vi "Tesina_Frullo_Corrado.vi"() -> ()   [LabVIEW 2021]
uses:
  <vilib>/express/express analysis/Spectral/XNode/ExpressSpectralMeasurementsBlockNode.xnode
  <vilib>/express/express analysis/Spectral/Block/exnSpectralBlock spectral measurements RMS poly.vi
  <vilib>/express/express analysis/Spectral/Block/exnSpectralBlock spectral measurements RMS array WFM.vi
  <vilib>/express/express analysis/Spectral/Block/exnSpectralBlock spectral measurements RMS DDT.vi
panel:
  in  "Lower Cut-Off (Hz)":dbl=100.0 caption="Lower Cut-Off"
  out "Originale":bool
  out "Filtrato":bool
  out "Caricamento...":i32(slide) scale=0.0..4.0
  in  "Vuoi ascoltare il campione filtrato?":bool
  out "FFT - (RMS) [filtrato]":dynamicdata(graph)
  out "Time-domain [filtrato]":dynamicdata(graph)
  in  "Vuoi filtrare il campione?":bool
  out "Quando il led si accende, preparati a registrare!":bool
  out "FFT - (RMS)":cluster{"f0":dbl, "df":dbl, "magnitude":dbl[]}[](graph)
  out "Time-domain":waveform(dbl)[](graph)
  in  "Vuoi riascoltare il campione caricato?":bool
  in  "Carica file da analizzare [.wav]":path
  in  "1) Vuoi registrare un campione o analizzarne uno già salvato?":bool
  in  "Salva file [.wav]":path
  in  "Vuoi salvare il campione acquisito?":bool
  in  "Duration (s)":dbl=1.0
  in  "Sample rate (Hz)":dbl=22050.0
  in  "Vuoi riprodurre il campione acquisito?":bool
  out "Inizio registrazione":bool
  out "Fine registrazione":bool
  out "Salvato":bool
  # "REGISTRA E ANALIZZA"
  # "ANALIZZA"
  # "Se vuoi registrare un nuovo campione, salta questo passaggio e procedi con le FASI 2 e 3"
  # "Se vuoi analizzare un campione già acquisito, selezionalo qua (poi passa direttamente alla FASE 4):"
  # "Le FASI 2 e 3 sono da considerare SOLO SE si vuole registrare un nuovo campione, ricorda di specificare ogni parametro (compreso il nome del file) prima dell'esecuzione"
  # "2) FASE DI ACQUISIZIONE: imposta durata e sample rate del segnale"
  # "NO"
  # "SI"
  # "3) SALVATAGGIO"
  # "NO"
  # "SI"
  # "PERCORSO DI DEFAULT"
  # "C:\\Users\\alefr\\Dropbox\\Uni\\Misure\\tesina misure\\sample\\**NOME DEL FILE**.wav"
  # "4) FASE DI ANALISI"
  # "NO"
  # "SI"
  # "E' in riproduzione il segnale:"
  # "NO"
  # "SI"
  # "NO"
  # "SI"
  # "GRAFICI DEL SEGNALE FILTRATO"
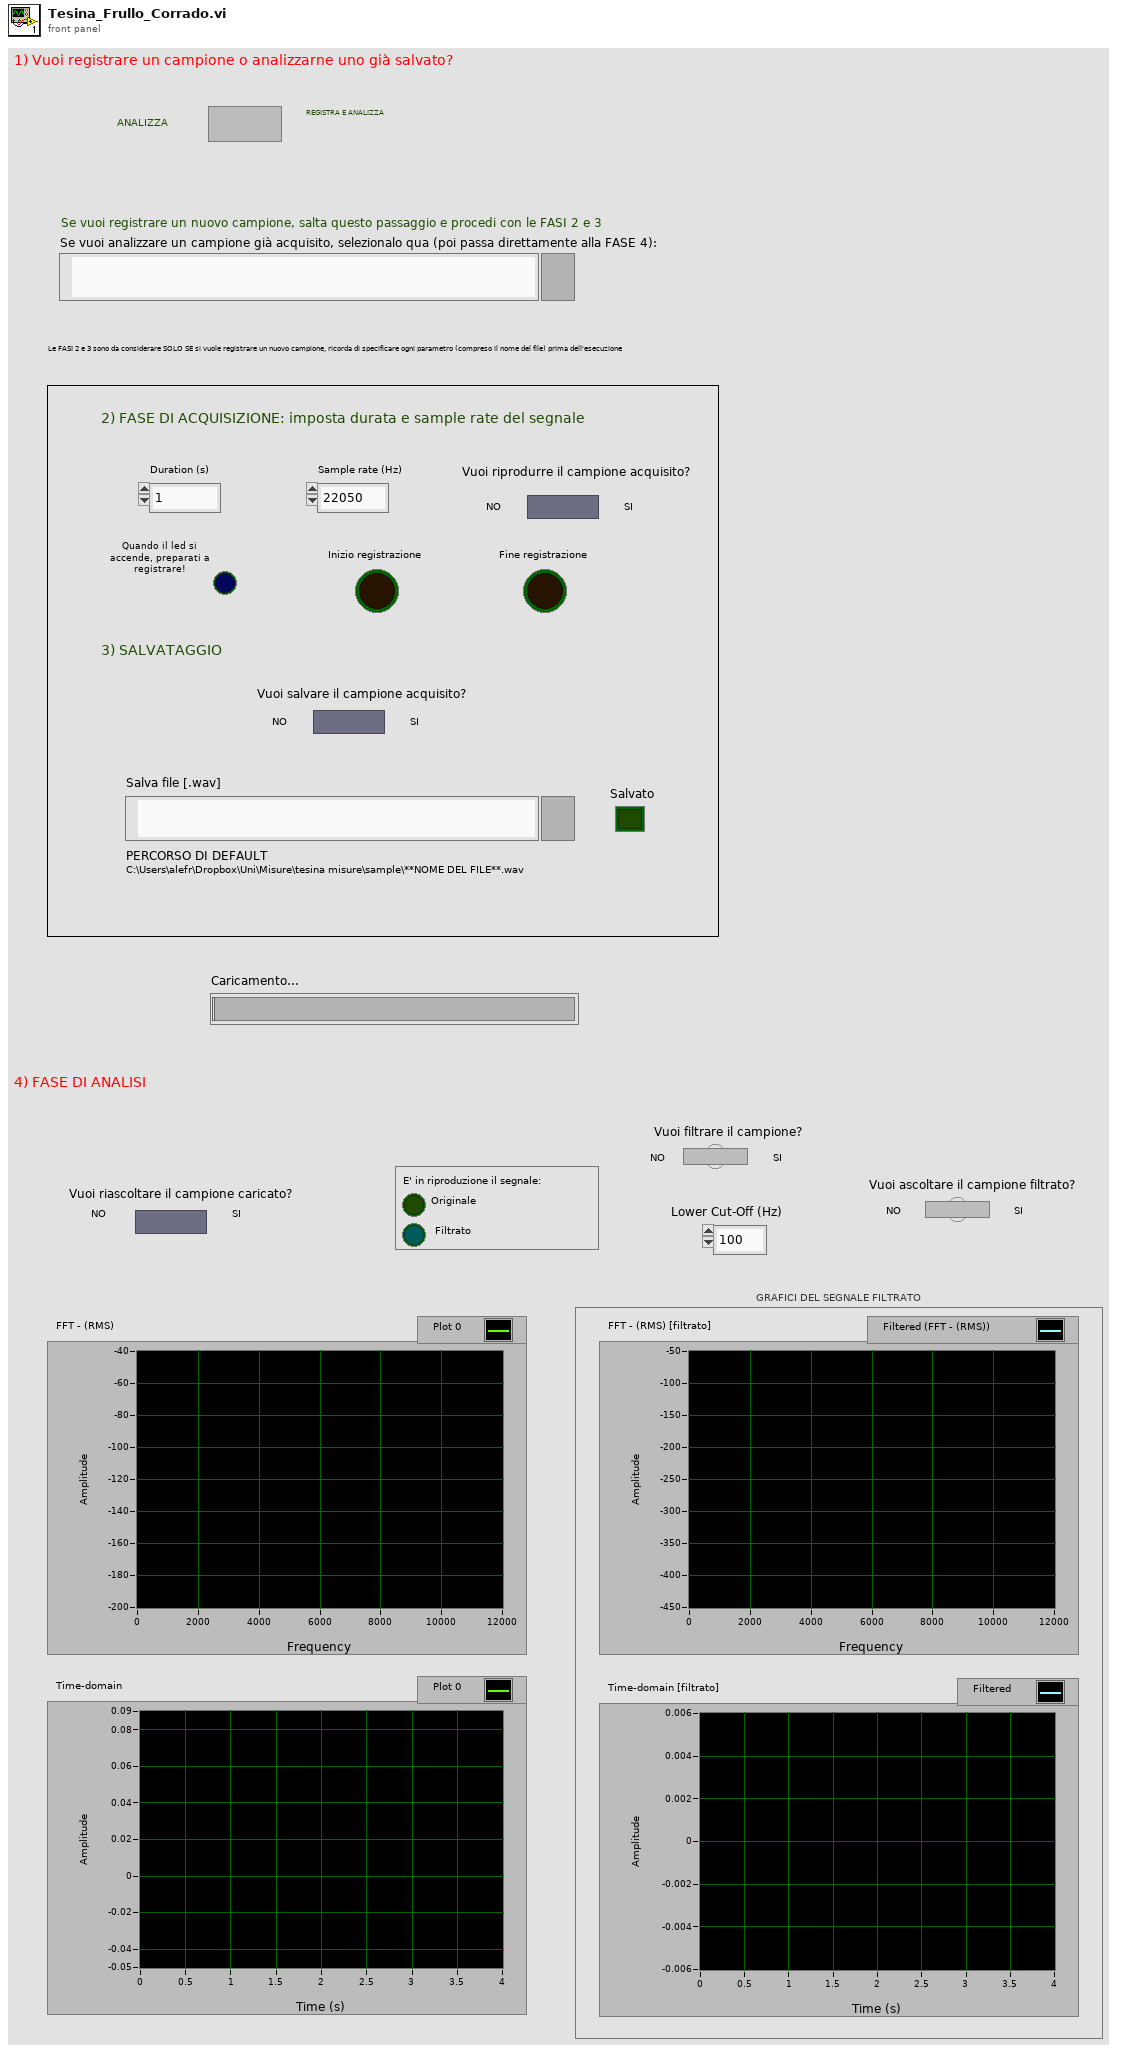
[diagram p1: front panel]
types:
  T1 = cluster{"averaging mode":u16, "weighting mode":u16, "number of averages":u32}
  T2 = cluster{"dB On (F)":bool, "unwrap phase (F)":bool, "convert to degree (F)":bool}
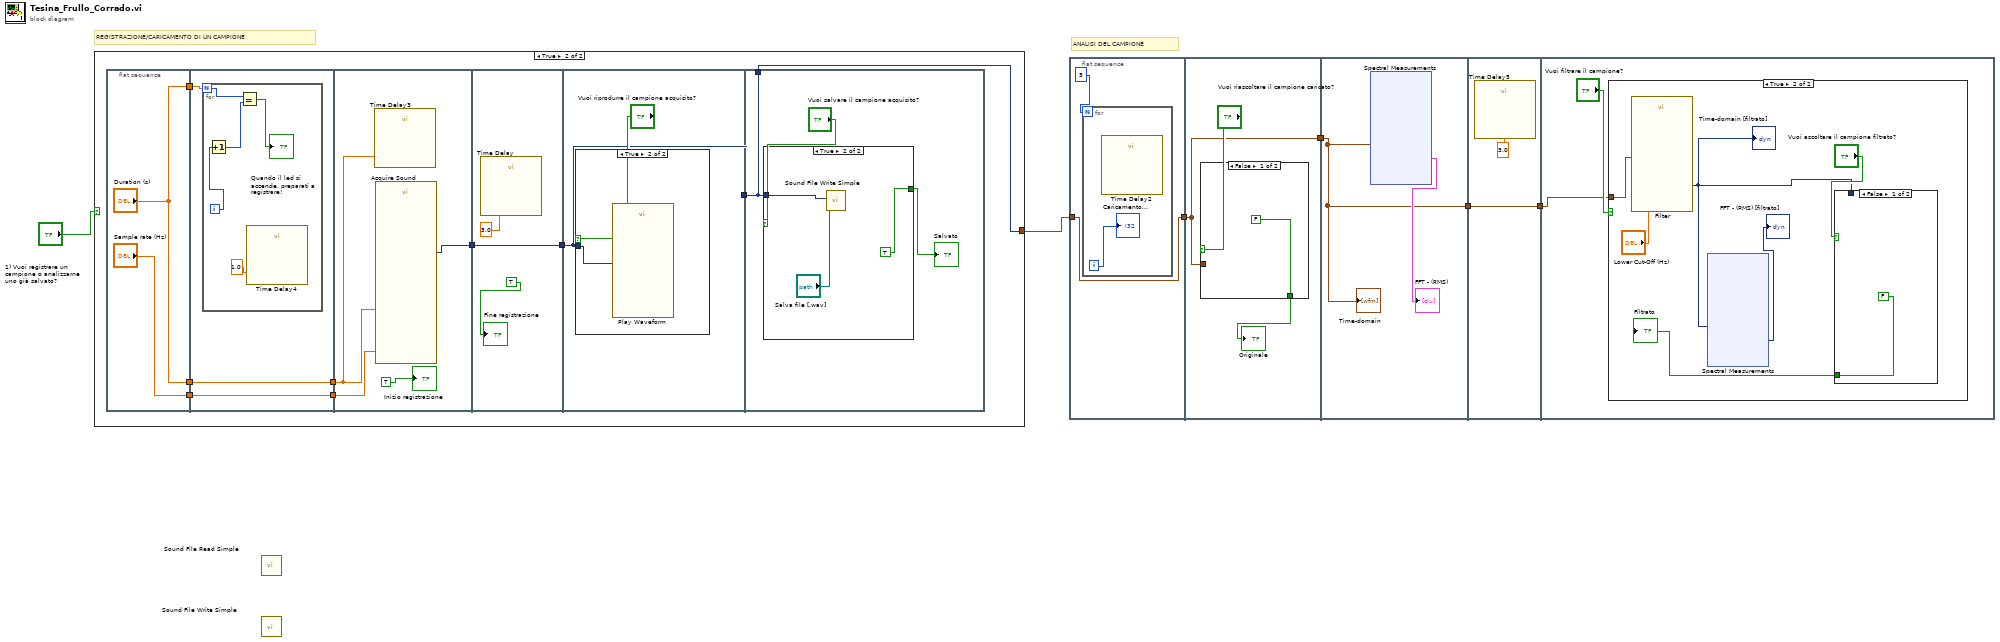
[diagram p0: block diagram]
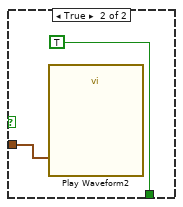
[diagram p2: hidden frame]
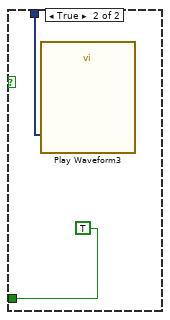
[diagram p4: hidden frame]
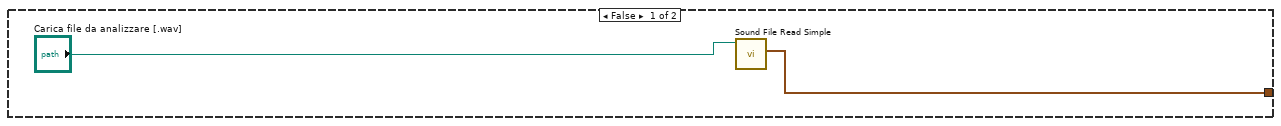
[diagram p5: hidden frame]
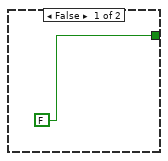
[diagram p7: hidden frame]
diagram:
  # "ANALISI DEL CAMPIONE"
  # "REGISTRAZIONE/CARICAMENTO DI UN CAMPIONE"
  n1 = case shown="True" "1) Vuoi registrare un campione o analizzarne uno già salvato?" {
    tunnel: [w7 w14] -> w5
    frame False {
      n2 = call <vilib>:"Sound File Read Simple.vi"("path"="Carica file da analizzare [.wav]") -> ("data"=w7:waveform(dbl)[])  [unwired: 7 in, 3 out]
    }
    frame True {
      n3 = flat-sequence {
        tunnel: ["Sample rate (Hz)"] -> w13
        tunnel: ["Duration (s)"] -> w11
        tunnel: ["Duration (s)"] -> w9
        tunnel: w13 -> [w22]
        tunnel: [w22] -> w12
        tunnel: w11 -> [w21]
        tunnel: [w21] -> w10
        tunnel: w9 -> [w20]
        tunnel: w12 -> [w30]
        tunnel: w10 -> [w29]
        tunnel: [w28] -> w17
        tunnel: [w32] -> w16
        tunnel: w17 -> [w32]
        tunnel: w16 -> [w35]
        tunnel: [w35] -> w15
        tunnel: w15 -> [w39]
        tunnel: [w39] -> w14
        frame #0 {
        }
        frame #1 {
          n4 = for {
            N: w20 -> [w27]
            i -> [w26]
            n5 = Increment(x=w26) -> (x+1=w25:i32)
            n6 = Equal?(x=w27, y=w25) -> (x = y?=→"Quando il led si accende, preparati a registrare!":bool)
            n7 = call "Time Delay4"("Delay Time (s)"=1.0) -> ()  [unwired: 10 in, 1 out]
          }
        }
        frame #2 {
          n8 = call "Time Delay3"("Delay Time (s)"=w29) -> ()  [unwired: 10 in, 1 out]
          n9 = call "Acquire Sound"("Duration (s)"=w29, "Sample rate (Hz)"=w30) -> ("Data"=w28:dynamicdata)  [unwired: 16 in, 1 out]
          "Inizio registrazione" <- TRUE ("Acquisito")
        }
        frame #3 {
          n10 = call "Time Delay"("Delay Time (s)"=3.0) -> ()  [unwired: 10 in, 1 out]
          "Fine registrazione" <- TRUE ("Inizio registrazione 2")
        }
        frame #4 {
          n11 = case shown="True" "Vuoi riprodurre il campione acquisito?" {
            tunnel: w35 -> [_ w37]
            frame False {
            }
            frame True {
              n12 = call "Play Waveform"("Data"=w37) -> ()  [unwired: 18 in, 1 out]
            }
          }
        }
        frame #5 {
          n13 = case shown="True" "Vuoi salvare il campione acquisito?" {
            tunnel: w39 -> [_ w44]
            tunnel: [FALSE TRUE ("Acquisito")] -> w38
            frame False {
            }
            frame True {
              n14 = call <vilib>:"Sound File Write Simple.vi"("data"=w44, "path"="Salva file [.wav]") -> ()  [unwired: 8 in, 2 out]
            }
          }
          "Salvato" <- w38
        }
      }
    }
  }
  n15 = call <vilib>:"Sound File Read Simple.vi"() -> ()  [unwired: 8 in, 4 out]
  n16 = call <vilib>:"Sound File Write Simple.vi"() -> ()  [unwired: 10 in, 2 out]
  n17 = flat-sequence {
    tunnel: w5 -> [w46]
    tunnel: [w46] -> w3
    tunnel: [w49] -> w4
    tunnel: w3 -> [w49]
    tunnel: w4 -> [w54]
    tunnel: [w54] -> w2
    tunnel: w2 -> [w67]
    tunnel: [w67] -> w1
    tunnel: w1 -> [w68]
    frame #0 {
      n18 = for {
        N: 5 -> [_]
        i -> [w47]
        n19 = call "Time Delay2"() -> ()  [unwired: 11 in, 1 out]
        "Caricamento..." <- w47
      }
    }
    frame #1 {
      n20 = case shown="False" "Vuoi riascoltare il campione caricato?" {
        tunnel: w49 -> [_ w53]
        tunnel: [FALSE TRUE ("Originale")] -> w48
        frame False {
        }
        frame True {
          n21 = call "Play Waveform2"("Data"=w53) -> ()  [unwired: 18 in, 1 out]
        }
      }
      "Originale" <- w48
    }
    frame #2 {
      n22 = xnode "Spectral Measurements"("Signals"=w54) -> ("FFT - (RMS)"=→"FFT - (RMS)":cluster{"f0":dbl, "df":dbl, "magnitude":dbl[]}[])  [unwired: 1 in, 2 out]
      "Time-domain" <- w54
    }
    frame #3 {
      n23 = call "Time Delay5"("Delay Time (s)"=3.0) -> ()  [unwired: 10 in, 1 out]
    }
    frame #4 {
      n24 = case shown="True" "Vuoi filtrare il campione?" {
        tunnel: w68 -> [_ w75]
        frame False {
        }
        frame True {
          n25 = call "Filter"("Lower Cut-Off"="Lower Cut-Off (Hz)", "Signal"=w75) -> ("Filtered Signal"=w72:dynamicdata)  [unwired: 8 in, 1 out]
          "Time-domain [filtrato]" <- w72
          n26 = xnode "Spectral Measurements"("Signals"=w72) -> ("FFT - (RMS)"=→"FFT - (RMS) [filtrato]":dynamicdata)  [unwired: 1 in, 2 out]
          n27 = case shown="False" "Vuoi ascoltare il campione filtrato?" {
            tunnel: w72 -> [_ w78]
            tunnel: [FALSE TRUE ("Filtrato")] -> w70
            frame False {
            }
            frame True {
              n28 = call "Play Waveform3"("Data"=w78) -> ()  [unwired: 18 in, 1 out]
            }
          }
          "Filtrato" <- w70
        }
      }
    }
  }
